vi "RSZVB Write Source Power Correction Data.vi"(5 "Calibrated Wave":string, 6 "Power Correction Values":dbl[](array[numeric]) format="%^.3e", 7 "Number Of Values (1)":i32=1, 8 "error in (no error)":errorcluster {"code" format="%.0x"}, 9 "Port Number (1)":i32=1, 10 "Channel (1)":i32=1, 11 "VISA session":refnum<visa-resource-name>) -> (0 "error out":errorcluster {"code" format="%.0x"}, 3 "dup VISA session":refnum<visa-resource-name>)   [LabVIEW 2011]
doc: "This VI writes source power correction data sets. \n\nNote(s):\n\n(1) A power correction data set contains n real values. Each value corresponds to the ratio of the actual power at the reference plane (value provided by the used source) to the uncalibrated power in dB. \n\n(2) The number n is equal to the number of sweep points.\n\n(3) Writing correction data fails if the number of transferred values is not equal to the number of sweep points.\n \n\nRemote-control command(s):\nSOURce<Ch>:POWer<Pt>:CORRection:DATA '<src_string>', <numeric_value>..."
uses:
  _utility/RSZVB Global Data.vi
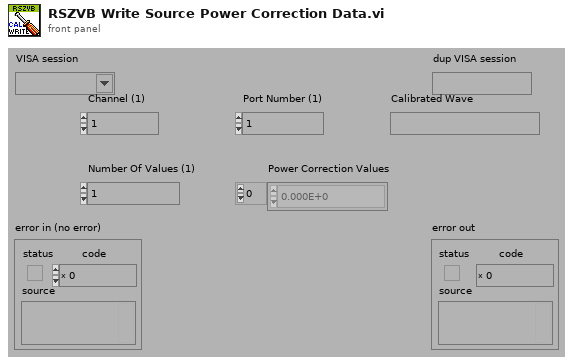
[diagram p1: front panel]
types:
  T1 = cluster{"Error Checking (T: On)":bool, "Installed Options":string[], "Data Valid?":bool, "Ports":i32, "Model":string[], "Option Checking (T: On)":bool}[]
  T2 = cluster{"Error Checking (T: On)":bool, "Installed Options":string[], "Data Valid?":bool, "Ports":i32, "Model":string[], "Option Checking (T: On)":bool}
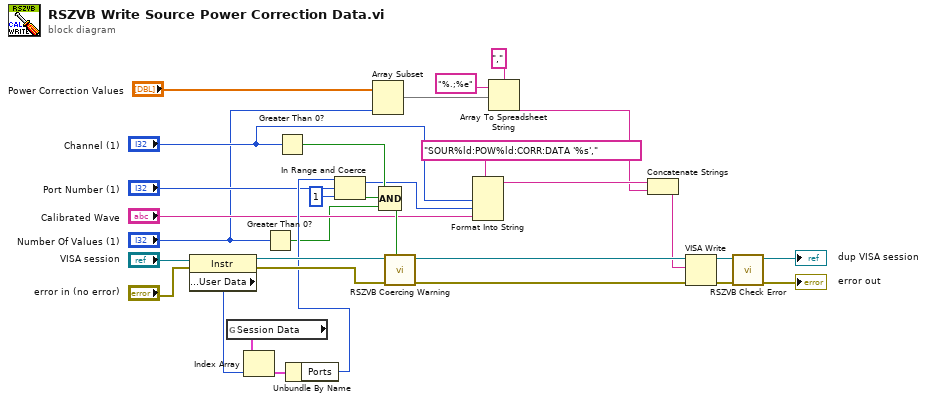
[diagram p0: block diagram]
diagram:
  n1 = property class="Instr"(reference="VISA session", error in="error in (no error)") -> (reference out=w24:refnum<visa-resource-name>, error out=w25:errorcluster, "General Settings:User Data"=w26:u32)
  n2 = global read "RSZVB Global Data.vi" "Session Data"() -> (w27:T1)
  n3 = Index Array(array=w27, index=w26) -> (element=w28:T2)
  n4 = Greater Than 0?(x="Number Of Values (1)") -> (x > 0?=w9:bool)
  n5 = Greater Than 0?(x="Channel (1)") -> (x > 0?=w30:bool)
  n6 = Unbundle By Name(w28) -> ("Ports"=w22:i32)
  n7 = In Range and Coerce(upper limit=w22, x="Port Number (1)", lower limit=1) -> (coerced(x)=w19:i32, In Range?=w21:bool)
  n8 = Array Subset(array="Power Correction Values", length="Number Of Values (1)") -> (w2:dbl[])  [unwired: 1 in]
  n9 = Compound Arithmetic op=AND(w30, w21, w9) -> (w29:bool)
  n10 = call "RSZVB Coercing Warning.vi"("In Range?"=w29, "error in (no error)"=w25, "VISA session"=w24) -> ("error out"=w31:errorcluster, "dup VISA session"=w32:refnum<visa-resource-name>)  [unwired: 7 in]
  n11 = Format Into String(format string="SOUR%ld:POW%ld:CORR:DATA '%s',", "Channel (1)", w19, "Calibrated Wave") -> (resulting string=w7:string)  [unwired: 2 in, 1 out]
  n12 = Array To Spreadsheet String(delimiter (Tab)=",", array=w2, 3:"%.;%e") -> (spreadsheet string=w4:string)
  n13 = Concatenate Strings(w7, w4) -> (w6:string)
  n14 = VISA Write(VISA resource name=w32, write buffer=w6, error in (no error)=w31) -> (VISA resource name out=w15:refnum<visa-resource-name>, error out=w16:errorcluster)  [unwired: 1 out]
  n15 = call "RSZVB Check Error.vi"("error in (no error)"=w16, "VISA session"=w15) -> ("error out"=→"error out":errorcluster, "dup VISA session"=→"dup VISA session":refnum<visa-resource-name>)  [unwired: 8 in]
